vi "Lift Globals.vi"() -> ()   [LabVIEW 2017]
uses:
  Lift Notifier.ctl
  Lift Control Type.ctl
  Lift Enum States.ctl
panel:
  out "Load":bool
  out "Reset":bool
  in  "Lift Cals":dbl[](array[numeric])
  in  "Lift Position":i32
  out "Lift Lower Switch":bool
  out "Lift Upper Switch":bool
  in  "Lift Execute Notifier":refnum<notifier>
  in  "Lift Set Notifier":refnum<notifier>
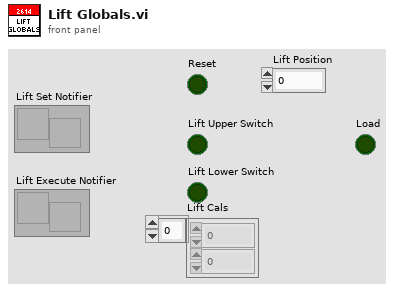
[diagram p1: front panel]
diagram:
